vi "RT Main.vi"() -> ()   [LabVIEW 2014]
uses:
  <vilib>/myRIO/Instrument Drivers/Utilities/Utilities.lvlib
  <vilib>/myRIO/Express VI/Onboard IO/AI/AI Express VI.xnode
  <vilib>/myRIO/Instrument Drivers/Onboard IO/AI/vis/Read.vi
  <vilib>/myRIO/Instrument Drivers/Onboard IO/AI/AI.lvlib
  <vilib>/myRIO/Common/Instrument Driver Framework/Utilities/typedefs/Analog Scaling Constants.ctl
  <vilib>/myRIO/Common/Instrument Driver Framework/Utilities/typedefs/Analog Scaling Constants List.ctl
  <vilib>/myRIO/Common/Instrument Driver Framework/myRIO v1.0/AI/typedefs/AI Channels Enum.ctl
  <vilib>/myRIO/Common/Instrument Driver Framework/myRIO v1.0/AI/typedefs/AI Channels List.ctl
  <vilib>/myRIO/Common/Instrument Driver Framework/Utilities/typedefs/Generic FPGA Reference.ctl
  <vilib>/myRIO/Common/Instrument Driver Framework/Utilities/typedefs/myRIO v1.0 Reference.ctl
  <vilib>/myRIO/Common/Instrument Driver Framework/Utilities/typedefs/Hardware Version Enum.ctl
  <vilib>/myRIO/Common/Instrument Driver Framework/Utilities/typedefs/myRIO Generic Hardware Reference.ctl
  <vilib>/myRIO/Instrument Drivers/Onboard IO/AI/typedefs/AI Reference.ctl
  <vilib>/myRIO/Instrument Drivers/Onboard IO/AI/vis/myRIO AI Open.xnode
  <vilib>/myRIO/Common/Instrument Driver Framework/Utilities/vis/Is FPGA Ref Available.vi
  <vilib>/userdefined/High Color/nirio_resource_hc.ctl
  <vilib>/myRIO/Express VI/Onboard IO/Encoder/Encoder Express VI.xnode
  <vilib>/myRIO/Instrument Drivers/Onboard IO/Encoder/vis/Read.vi
  <vilib>/myRIO/Instrument Drivers/Onboard IO/Encoder/Encoder.lvlib
  <vilib>/myRIO/Common/Instrument Driver Framework/myRIO v1.0/Encoder/typedefs/Encoder Signal Mode.ctl
  <vilib>/myRIO/Common/Instrument Driver Framework/myRIO v1.0/Encoder/typedefs/Encoder Channels Enum.ctl
  <vilib>/myRIO/Instrument Drivers/Onboard IO/Encoder/typedefs/Encoder Reference.ctl
  <vilib>/myRIO/Instrument Drivers/Onboard IO/Encoder/vis/myRIO Encoder Open.xnode
  <vilib>/myRIO/Common/Instrument Driver Framework/myRIO v1.0/AI/vis/myRIO v1.1 Open AI.vi
  <vilib>/myRIO/Common/Instrument Driver Framework/myRIO v1.0/Encoder/vis/myRIO v1.1 Open Encoder.vi
  <vilib>/myRIO/Common/Instrument Driver Framework/myRIO v1.0/Encoder/vis/myRIO v1.0 Configure Encoder.vi
  <vilib>/myRIO/Common/Instrument Driver Framework/myRIO v1.0/Encoder/typedefs/Encoder Configuration v1.0.ctl
  <vilib>/myRIO/Express VI/Onboard IO/PWM/PWM Express VI.xnode
  <vilib>/myRIO/Instrument Drivers/Onboard IO/PWM/vis/Set Duty Cycle and Frequency.vi
  <vilib>/myRIO/Instrument Drivers/Onboard IO/PWM/PWM.lvlib
  <vilib>/myRIO/Instrument Drivers/Onboard IO/PWM/typedefs/PWM Configuration.ctl
  <vilib>/myRIO/Common/Instrument Driver Framework/myRIO v1.0/PWM/typedefs/PWM Channels Enum.ctl
  <vilib>/myRIO/Instrument Drivers/Onboard IO/PWM/typedefs/PWM Reference.ctl
  <vilib>/myRIO/Instrument Drivers/Onboard IO/PWM/vis/myRIO PWM Open.xnode
  <vilib>/myRIO/Common/Instrument Driver Framework/myRIO v1.0/PWM/vis/myRIO v1.1 Open PWM.vi
  <vilib>/myRIO/Express VI/Onboard IO/DO/DO Express VI.xnode
  <vilib>/myRIO/Instrument Drivers/Onboard IO/DIO/vis/Write.vi
  <vilib>/myRIO/Instrument Drivers/Onboard IO/DIO/DIO.lvlib
  <vilib>/myRIO/Common/Instrument Driver Framework/myRIO v1.0/DIO/typedefs/DIO Channels Enum.ctl
  <vilib>/myRIO/Common/Instrument Driver Framework/myRIO v1.0/DIO/typedefs/DIO Channels List.ctl
  <vilib>/myRIO/Instrument Drivers/Onboard IO/DIO/typedefs/DIO Reference.ctl
  <vilib>/myRIO/Instrument Drivers/Onboard IO/DIO/vis/myRIO DIO Open.xnode
  <vilib>/myRIO/Common/Instrument Driver Framework/myRIO v1.0/DIO/vis/myRIO v1.1 Open DIO.vi
panel:
  out "Encoder Count":i32
  out "IR Sensor Output":dbl(graph)
  in  "Stop Button":bool
  # "Rover Demo (Real Time)"
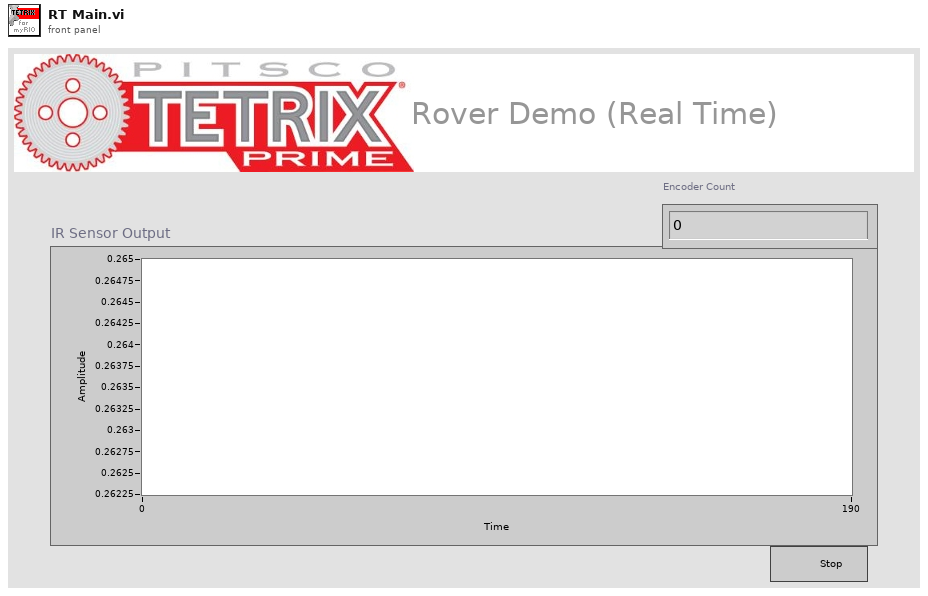
[diagram p1: front panel]
types:
  T1 = typedef "DIO.lvlib/DIO Reference.ctl" = cluster{"myRIO Reference":T2, "DIO Channels List":T6}
  T2 = typedef "myRIO Generic Hardware Reference.ctl" = cluster{"myRIO Model":T3, "myRIO Hardware Reference":T4}
  T3 = typedef "Hardware Version Enum.ctl" = enum16{"Unknown", "myRIO-1900", "myRIO-1950"}
  T4 = typedef "myRIO v1.0 Reference.ctl" = cluster{"Generic FPGA Reference":T5, "Allow multiple opens":bool}
  T5 = typedef "Generic FPGA Reference.ctl" = refnum<k20>
  T6 = typedef "DIO Channels List.ctl" = T7[]
  T7 = typedef "DIO Channels Enum.ctl" = enum16{"Not Connected", "C/DIO0", "C/DIO1", "C/DIO2", "C/DIO3", "C/DIO4", "C/DIO5", "C/DIO6", "C/DIO7", "A/DIO0", "A/DIO1", "A/DIO2", "A/DIO3", "A/DIO4", "A/DIO5", "A/DIO6", "A/DIO7", "A/DIO8", "A/DIO9", "A/DIO10", "A/DIO11", "A/DIO12", "A/DIO13", "A/DIO14", "A/DIO15", "B/DIO0", "B/DIO1", "B/DIO2", "B/DIO3", "B/DIO4", "B/DIO5", "B/DIO6", "B/DIO7", "B/DIO8", "B/DIO9", "B/DIO10", "B/DIO11", "B/DIO12", "B/DIO13", "B/DIO14", "B/DIO15", "LED0", "LED1", "LED2", "LED3", "Button0"}
  T8 = typedef "nirio_resource_hc.ctl" = tag
  T9 = typedef "PWM.lvlib/PWM Reference.ctl" = cluster{"myRIO Reference":T2, "PWM Channels Enum":T10, "PWM Configuration":T11}
  T10 = typedef "PWM Channels Enum.ctl" = enum16{"Not Connected", "C/PWM0", "C/PWM1", "A/PWM0", "A/PWM1", "A/PWM2", "B/PWM0", "B/PWM1", "B/PWM2"}
  T11 = typedef "PWM.lvlib/PWM Configuration.ctl" = cluster{"Frequency":dbl, "Duty Cycle":dbl}
  T12 = typedef "Encoder.lvlib/Encoder Reference.ctl" = cluster{"myRIO Reference":T2, "Encoder Channels Enum":T13}
  T13 = typedef "Encoder Channels Enum.ctl" = enum16{"Not Connected", "C/ENC0", "C/ENC1", "A/ENC", "B/ENC"}
  T14 = typedef "Encoder Signal Mode.ctl" = enum16{"Quadrature phase signal", "Step and direction signal"}
  T15 = typedef "AI.lvlib/AI Reference.ctl" = cluster{"myRIO Reference":T2, "AI Channels List":T16, "AI Scaling Constants List":T18}
  T16 = typedef "AI Channels List.ctl" = T17[]
  T17 = typedef "AI Channels Enum.ctl" = enum16{"Not Connected", "AudioIn/Left", "AudioIn/Right", "C/AI0", "C/AI1", "A/AI0", "A/AI1", "A/AI2", "A/AI3", "B/AI0", "B/AI1", "B/AI2", "B/AI3"}
  T18 = typedef "Analog Scaling Constants List.ctl" = T19[]
  T19 = typedef "Analog Scaling Constants.ctl" = cluster{"LSB Weight (Volts)":dbl, "Offset (Volts)":dbl, "Signed?":bool}
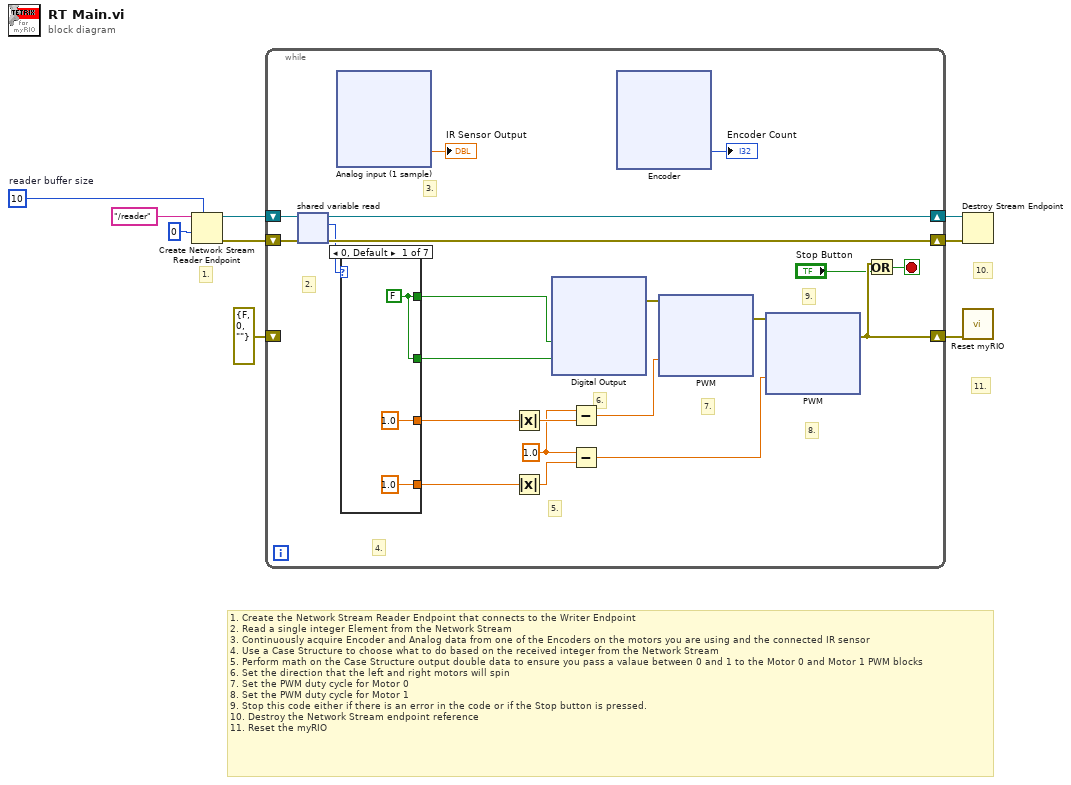
[diagram p0: block diagram]
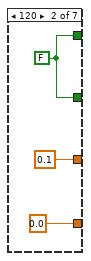
[diagram p2: hidden frame]
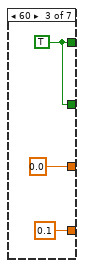
[diagram p3: hidden frame]
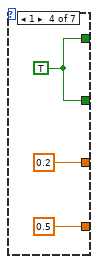
[diagram p4: hidden frame]
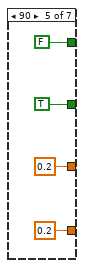
[diagram p5: hidden frame]
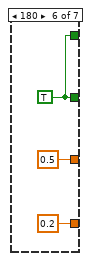
[diagram p6: hidden frame]
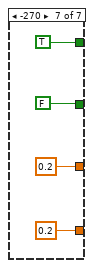
[diagram p7: hidden frame]
diagram:
  w7 = 10  # reader buffer size
  # "1. Create the Network Stream Reader Endpoint that connects to the Writer Endpoint\n2. Read a single integer Element from the Network Stream \n3. Continuously acquire Encoder and Analog data from one of the Encoders on the motors you are using and the connected IR sensor\n4. Use a Case Structure to choose what to do based on the received integer from the Network Stream\n5. Perform math on the Case Structure output double data to ensure you pass a valaue between 0 and 1 to the Motor 0 and Motor 1 PWM blocks \n6. Set the direction that the left and right motors will spin\n7. Set the PWM duty cycle for Motor 0\n8. Set the PWM duty cycle for Motor 1\n9. Stop this code either if there is an error in the code or if the Stop button is pressed.\n10. Destroy the Network Stream endpoint reference\n11. Reset the myRIO"
  # "11."
  # "10."
  # "1."
  n1 = Create Network Stream Reader Endpoint(7:w7, 9:0, 11:"/reader" ("reader name")) -> (0:w4:errorcluster, 3:w5:refnum<k21>)  [unwired: 4 in]
  n2 = while {
    shift-right: [w25] -> w8
    shift-left: errorcluster {"status"=FALSE, "code"=0, "source"=""} ("error in (no error)") -> [_]
    shift-right: [w16] -> w3
    shift-left: w5 -> [w18]
    shift-right: [w15] -> w2
    shift-left: w4 -> [w17]
    stop <- w26 stop-if-true
    w19 = 1.0 ("x")
    # "9."
    # "8."
    # "6."
    # "7."
    # "5."
    # "4."
    # "2."
    # "3."
    n3 = shared-variable-read(w18, w17) -> (w16:refnum<k21>, w15:errorcluster, w14:i32)  [unwired: 1 in, 1 out]
    n4 = xnode "Analog input (1 sample)"() -> ("B/AI0 (Pin 3)"=→"IR Sensor Output":dbl)  [unwired: 1 in, 1 out]
    n5 = case shown="0, Default" w14 {
      tunnel: [1.0 ("Motor 1") 0.1 ("Motor 1") 0.0 ("Motor 1") 0.2 ("Motor 1") 0.2 ("Motor 1") 0.5 ("Motor 1") 0.2 ("Motor 1")] -> w28
      tunnel: [1.0 ("Motor 1") 0.0 ("Motor 1") 0.1 ("Motor 1") 0.5 ("Motor 1") 0.2 ("Motor 1") 0.2 ("Motor 1") 0.2 ("Motor 1")] -> w27
      tunnel: [w220 w223 w226 w229 FALSE w236 TRUE] -> w11
      tunnel: [w220 w223 w226 w229 TRUE w236 FALSE] -> w10
      frame 0, Default {
        w220 = FALSE
      }
      frame 120 {
        w223 = FALSE
      }
      frame 60 {
        w226 = TRUE
      }
      frame 1 {
        w229 = TRUE
      }
      frame 90 {
      }
      frame 180 {
        w236 = TRUE
      }
      frame -270 {
      }
    }
    n6 = Absolute Value(x=w28) -> (abs(x)=w23:dbl)
    n7 = Absolute Value(x=w27) -> (abs(x)=w21:dbl)
    n8 = xnode "Digital Output"("M0 Dir (A/DIO2 (Pin 15))"=w11, "M1 Dir (A/DIO3 (Pin 17))"=w10) -> ("error out"=w30:errorcluster)  [unwired: 1 in]
    n9 = Subtract(x=w19, y=w23) -> (x-y=w22:dbl)
    n10 = Subtract(x=w19, y=w21) -> (x-y=w20:dbl)
    n11 = xnode "Encoder"() -> ("Counter Value"=→"Encoder Count":i32)  [unwired: 2 in, 3 out]
    n12 = xnode "PWM"("Duty Cycle"=w22, "error in (no error)"=w30) -> ("error out"=w29:errorcluster)
    n13 = xnode "PWM"("Duty Cycle"=w20, "error in (no error)"=w29) -> ("error out"=w25:errorcluster)
    n14 = Or(x=w25, y="Stop Button") -> (x .or. y?=w26:bool)
  }
  n15 = Destroy Stream Endpoint(8:w2, 11:w3) -> ()  [unwired: 1 out]
  n16 = call <vilib>:"Reset myRIO.vi"("error in (no error)"=w8) -> ()  [unwired: 10 in, 1 out]
